vi "SetOperationCycleEndTime.vi"(8 "error in":errorcluster, 10 "OperationRunEndTime":timestamp, 11 "OperationCycle in":refnum<class "OperationCycle.lvclass">) -> (0 "error out":errorcluster, 3 "OperationCycle out":refnum<class "OperationCycle.lvclass">)   [LabVIEW 2021, in "ProligentXMLGenerator.lvlib" / "OperationCycle.lvclass"]
doc: "Defines the end date of the operation run. If 'OperationStatus' is equal to 'NOT_COMPLETED' this value must be ommited. This value must be greater or equal than OperationRunEndTime.\n\nNote that the if the Data Warehouse already contains this operation run but it is not already closed, the OperationRunEndTime written in the Data Warehouse will be set according to the following rule: OperationRunEndTime(in database) = OperationRunStartTime(in database) + (OperationRunEndTime(from xml) - OperationRunStartTime(from xml)).\n\nThis value is restricted to \"1900-01-01T00:00:00Z\" -\"2100-01-01T00:00:00Z\"."
uses:
  OperationCycle.lvclass
  OperationCycle.lvclass/OperationCycle.ctl
  Base/DateTime/DateTime.lvclass
  Base/ExecutionStatus/Value.ctl
  Base/ExecutionStatus/ExecutionStatus.lvclass
  Base/Attribute/Attribute.lvclass
  C:/Projects/proligent-xml-generator-labview/src/ProligentXMLGenerator/Base/Attribute/Attribute.lvclass
  C:/Projects/proligent-xml-generator-labview/src/ProligentXMLGenerator/Base/DateTime/DateTime.lvclass
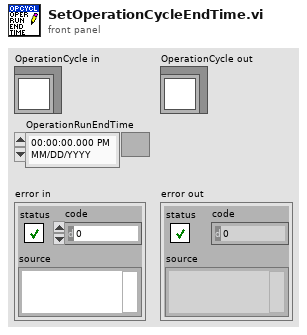
[diagram p1: front panel]
types:
  T1 = typedef "ProligentXMLGenerator.lvlib/ExecutionStatus.lvclass/Value.ctl" = enum16{"PASS", "FAIL", "NOT_COMPLETED", "ABORTED"}
  T2 = typedef "ProligentXMLGenerator.lvlib/OperationCycle.lvclass/Data.ctl" = cluster{"Name":string, "CustomData":refnum<class "CustomData.lvclass">, "ProcessFullName":refnum<class "ProcessFullName.lvclass">, "ProcessVersion":refnum<class "NonEmptyString_64.lvclass">, "OperationCycleId":refnum<class "Guid.lvclass">, "OperationName":refnum<class "NonEmptyString_65.lvclass">, "Location":refnum<class "FullName.lvclass">, "User":refnum<class "NonEmptyString_255.lvclass">, "OperationCycleStatus":refnum<class "ExecutionStatus.lvclass">, "OperationCycleStartTime":refnum<class "DateTime.lvclass">, "OperationCycleEndTime":refnum<class "DateTime.lvclass">, "TimeZoneInfoId":string}
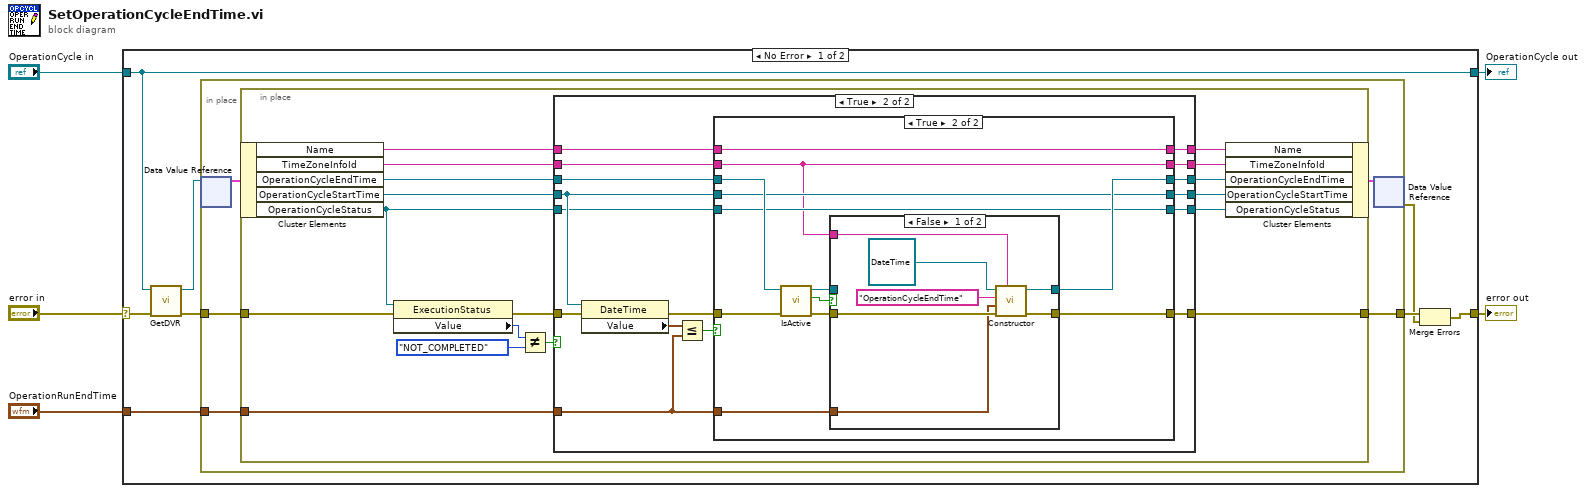
[diagram p0: block diagram]
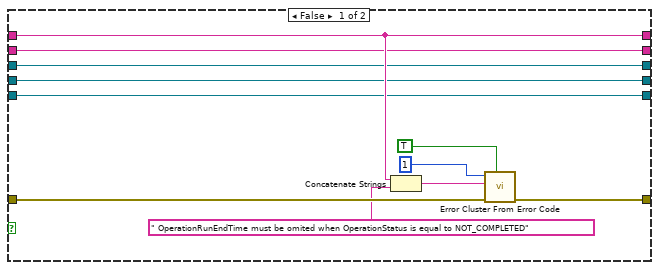
[diagram p2: hidden frame]
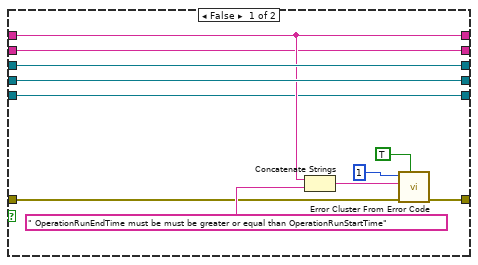
[diagram p3: hidden frame]
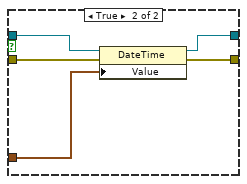
[diagram p4: hidden frame]
diagram:
  n1 = case shown="No Error" "error in" {
    selector: "error in" -> [w12 w98]
    tunnel: "OperationCycle in" -> [w7 w99]
    tunnel: [w9 w98] -> w3
    tunnel: "OperationRunEndTime" -> [w8 _]
    tunnel: [w7 w99] -> w1
    frame No Error {
      n2 = call "GetDVR.vi"("error in"=w12, "OperationCycle in"=w7) -> ("error out"=w11:errorcluster, "DVRReference"=w13:refnum<data-value>)  [unwired: 8 in]
      n3 = in-place "In Place Element Structure" {
        in-place-border: w11 -> [w16]
        in-place-border: [w18] -> w10
        in-place-border: w8 -> [w17]
        n4 = in-place-dvr #1(w13) -> (w15:T2)  [unwired: 1 out]
        n5 = in-place "In Place Element Structure" {
          in-place-border: [w35] -> w18
          in-place-border: w17 -> [w34]
          in-place-border: w16 -> [w33]
          n6 = in-place-cluster #2(w15) -> ("Name"=w26:string, "TimeZoneInfoId"=w19:string, "OperationCycleEndTime"=w27:refnum<class "DateTime.lvclass">, "OperationCycleStartTime"=w28:refnum<class "DateTime.lvclass">, "OperationCycleStatus"=w23:refnum<class "ExecutionStatus.lvclass">)
          n7 = property on="Property Node" class="ExecutionStatus"(reference=w23, error in=w33) -> (error out=w32:errorcluster, "Value"=w31:T1)  [unwired: 1 out]
          n8 = Not Equal?(x=w31, y=Value."NOT_COMPLETED") -> (x != y?=w29:bool)
          n9 = case shown="True" w29 {
            tunnel: [w43 w62] -> w35
            tunnel: w34 -> [_ w57]
            tunnel: w27 -> [w40 w61]
            tunnel: w32 -> [w44 w60]
            tunnel: w26 -> [w41 w55]
            tunnel: w28 -> [w39 w51]
            tunnel: [w40 w54] -> w25
            tunnel: [w41 w53] -> w24
            tunnel: w23 -> [w38 w50]
            tunnel: [w39 w52] -> w22
            tunnel: [w38 w49] -> w21
            tunnel: [w36 w48] -> w20
            tunnel: w19 -> [w36 w47]
            frame False {
              n10 = Concatenate Strings(w41, " OperationRunEndTime must be omited when OperationStatus is equal to NOT_COMPLETED" ("string")) -> (w45:string)
              n11 = call <vilib>:"Error Cluster From Error Code.vi"("show call chain? (False)"=TRUE, "error in (no error)"=w44, "error message (\"\")"=w45, "error code (0)"=1) -> ("error out"=w43:errorcluster)  [unwired: 5 in]
            }
            frame True {
              n12 = property on="Property Node" class="DateTime"(reference=w51, error in=w60) -> (error out=w59:errorcluster, "Value"=w58:timestamp)  [unwired: 1 out]
              n13 = Less Or Equal?(x=w58, y=w57) -> (x <= y?=w56:bool)
              n14 = case shown="True" w56 {
                tunnel: [w68 w85] -> w62
                tunnel: w61 -> [w67 w83]
                tunnel: w59 -> [w69 w81]
                tunnel: w57 -> [_ w80]
                tunnel: w55 -> [w65 w77]
                tunnel: [w67 w78] -> w54
                tunnel: [w65 w77] -> w53
                tunnel: [w66 w76] -> w52
                tunnel: w51 -> [w66 w76]
                tunnel: w50 -> [w64 w75]
                tunnel: [w64 w75] -> w49
                tunnel: [w63 w74] -> w48
                tunnel: w47 -> [w63 w74]
                frame False {
                  n15 = Concatenate Strings(w65, " OperationRunEndTime must be must be greater or equal than OperationRunStartTime" ("string")) -> (w71:string)
                  n16 = call <vilib>:"Error Cluster From Error Code.vi"("show call chain? (False)"=TRUE, "error in (no error)"=w69, "error message (\"\")"=w71, "error code (0)"=1) -> ("error out"=w68:errorcluster)  [unwired: 5 in]
                }
                frame True {
                  n17 = call "IsActive.vi"("error in"=w81, "Attribute in"=w83) -> ("error out"=w84:errorcluster, "IsActive"=w79:bool, "Attribute in"=w82:refnum<class "DateTime.lvclass">)  [unwired: 7 in]
                  n18 = case shown="False" w79 {
                    tunnel: [w91 w97] -> w85
                    tunnel: w80 -> [w88 w96]
                    tunnel: w84 -> [w92 w95]
                    tunnel: w82 -> [_ w94]
                    tunnel: [w87 w93] -> w78
                    tunnel: w74 -> [w86 _]
                    frame False {
                      n19 = call-dynamic "Constructor.vi"("TimeZoneInfoId"=w86, "error in"=w92, "Value"=w88, "Name"="OperationCycleEndTime", "DateTime in"=refnum<class "DateTime.lvclass"> refnum ("ProligentResultProcessor:DateTime")) -> ("error out"=w91:errorcluster, "DateTime out"=w87:refnum<class "DateTime.lvclass">)  [unwired: 5 in]
                    }
                    frame True {
                      n20 = property on="Property Node" class="DateTime"(reference=w94, error in=w95, "Value"=w96) -> (reference out=w93:refnum<class "DateTime.lvclass">, error out=w97:errorcluster)
                    }
                  }
                }
              }
            }
          }
          n21 = in-place-cluster #2("Name"=w24, "TimeZoneInfoId"=w20, "OperationCycleEndTime"=w25, "OperationCycleStartTime"=w22, "OperationCycleStatus"=w21) -> (w14:T2)
        }
        n22 = in-place-dvr #1(w14) -> (w6:errorcluster)  [unwired: 1 out]
      }
      n23 = Merge Errors(w10, w6) -> (w9:errorcluster)
    }
    frame Error {
    }
  }
  "error out" <- w3
  "OperationCycle out" <- w1
